vi "IQ to Mean Power.vi"(10 "Power Scaling":bool, 11 "IQ Data":dbl[](array[numeric])) -> (3 "Mean Power":dbl)   [LabVIEW 2021]
uses:
  <vilib>/Analysis/baseanly.llb/Mean (DBL).vi
  <vilib>/Analysis/NI_AALBase.lvlib
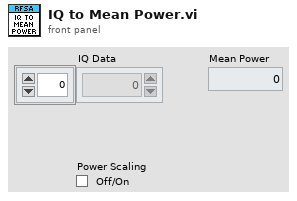
[diagram p1: front panel]
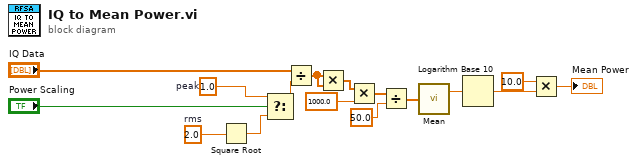
[diagram p0: block diagram]
diagram:
  w14 = 1.0  # peak
  w7 = 2.0  # rms
  n1 = Square Root(x=w7) -> (sqrt(x)=w15:dbl)
  n2 = Select(t=w14, s="Power Scaling", f=w15) -> (s? t:f=w8:dbl)
  n3 = Divide(x="IQ Data", y=w8) -> (x/y=w1:dbl[])
  n4 = Multiply(x=w1, y=w1) -> (x*y=w2:dbl[])
  n5 = Multiply(x=w2, y=1000.0) -> (x*y=w5:dbl[])
  n6 = Divide(x=w5, y=50.0) -> (x/y=w9:dbl[])
  n7 = call-poly <vilib>:"Mean.vi"("X"=w9) -> ("mean"=w10:dbl)  [unwired: 1 out]
  n8 = Logarithm Base 10(1:w10) -> (0:w11:dbl)
  n9 = Multiply(x=10.0, y=w11) -> (x*y=→"Mean Power":dbl)
